vi "Calculate single scan line duration.vi"(9 "Points in a scan line (~frame size)":i32, 11 "Dwell time (us)":dbl) -> (3 "Line scan time (us)":dbl)   [LabVIEW 2020]
uses:
  Global Variables/General Globals.vi
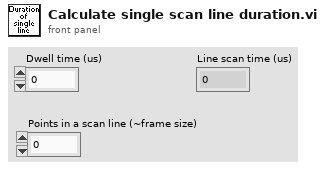
[diagram p1: front panel]
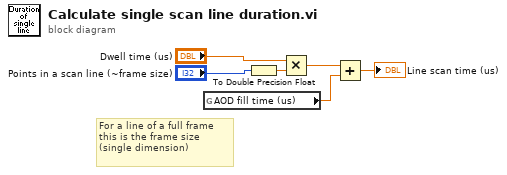
[diagram p0: block diagram]
diagram:
  # "For a line of a full frame this is the frame size (single dimension)"
  n1 = global read "General Globals.vi" "AOD fill time (us)"() -> (w1:dbl)
  n2 = To Double Precision Float(number="Points in a scan line (~frame size)") -> (double precision float=w5:dbl)
  n3 = Multiply(x="Dwell time (us)", y=w5) -> (x*y=w4:dbl)
  n4 = Add(x=w4, y=w1) -> (x+y=→"Line scan time (us)":dbl)
